vi "Main VI_1.vi"() -> ()   [LabVIEW 2024]
uses:
  Variable/Global.vi
  <vilib>/addons/database/Connection.llb/DB Tools Open Connec (String).vi
  <vilib>/addons/database/NI_Database_API.lvlib
  rpcrt4.dll
panel:
  out "String":string
  out "Config Path":path
  out "Communication error 3":bool
  out "Communication error 2":bool
  out "Communication error":bool
  in  "Logout 2":bool
  in  "USER TYPE":string(combo)="Admin"
  in  "USER NAME":string
  in  "PASSWORD":string
  in  "Login":bool
  out "Login Status":string
  in  "Calib":bool
  out "Login Type 2":string
  in  "Recipe":bool
  out "VER09042019":string
  out "Date Time":string
  in  "Manual":bool
  out "error out":errorcluster
  in  "Settings":bool
  in  "Report 2":bool
  in  "User_Setting":bool
  in  "Exit":bool
  in  "Run Test":bool
  out "User Name 2":string
  out "Login Type":string
  out "OK":bool
  # "TESTING DATALOGGING SYSTEM"
  # "31032025"
  # "SOFTWARE DEVELOPED BY:-SMOG Industries."
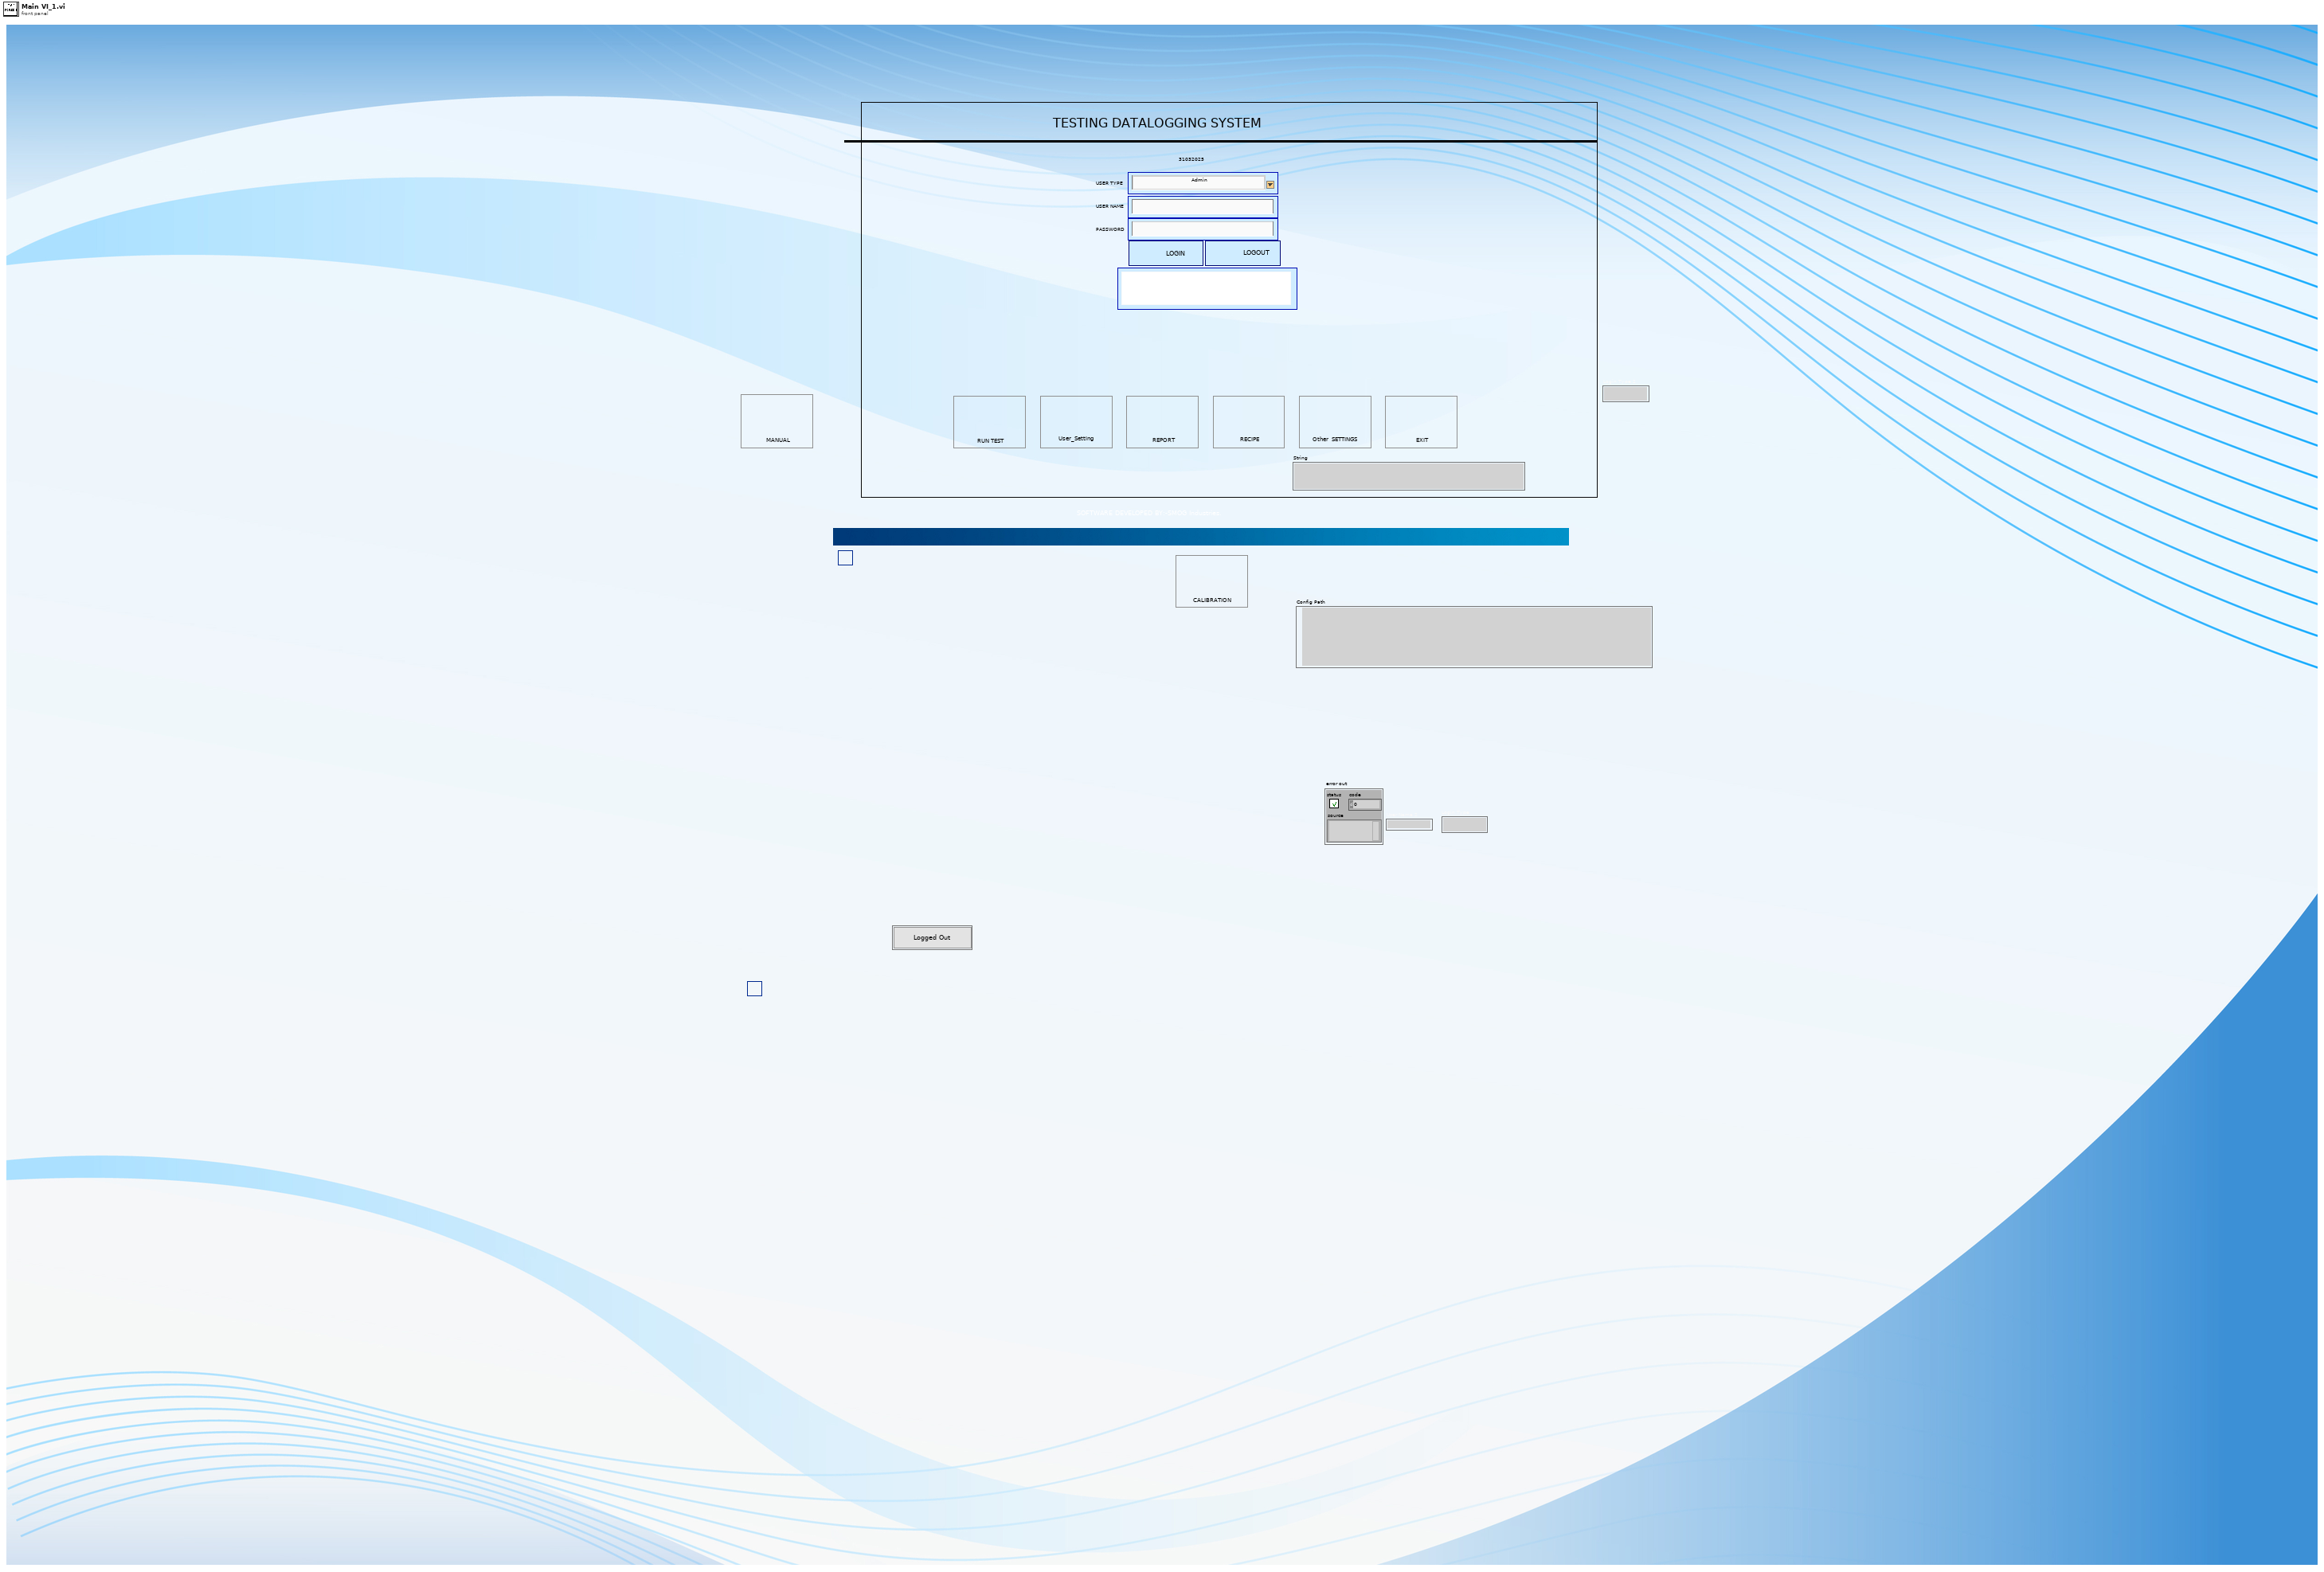
[diagram p1: front panel]
types:
  T1 = typedef "all path.ctl" = cluster{"User data":path, "Settings":path, "counter":path, "Test Setting":path, "IOs Path":path}
  T2 = enum16{"New barcode create", "barcode update", "check barcode", "database read", "barcode delete"}
  T3 = enum8{"Enabled", "Disabled", "Disabled and Grayed Out"}
  T4 = typedef "NI_Database_API.lvlib/Conn ObjectReference.ctl" = refnum<k1>
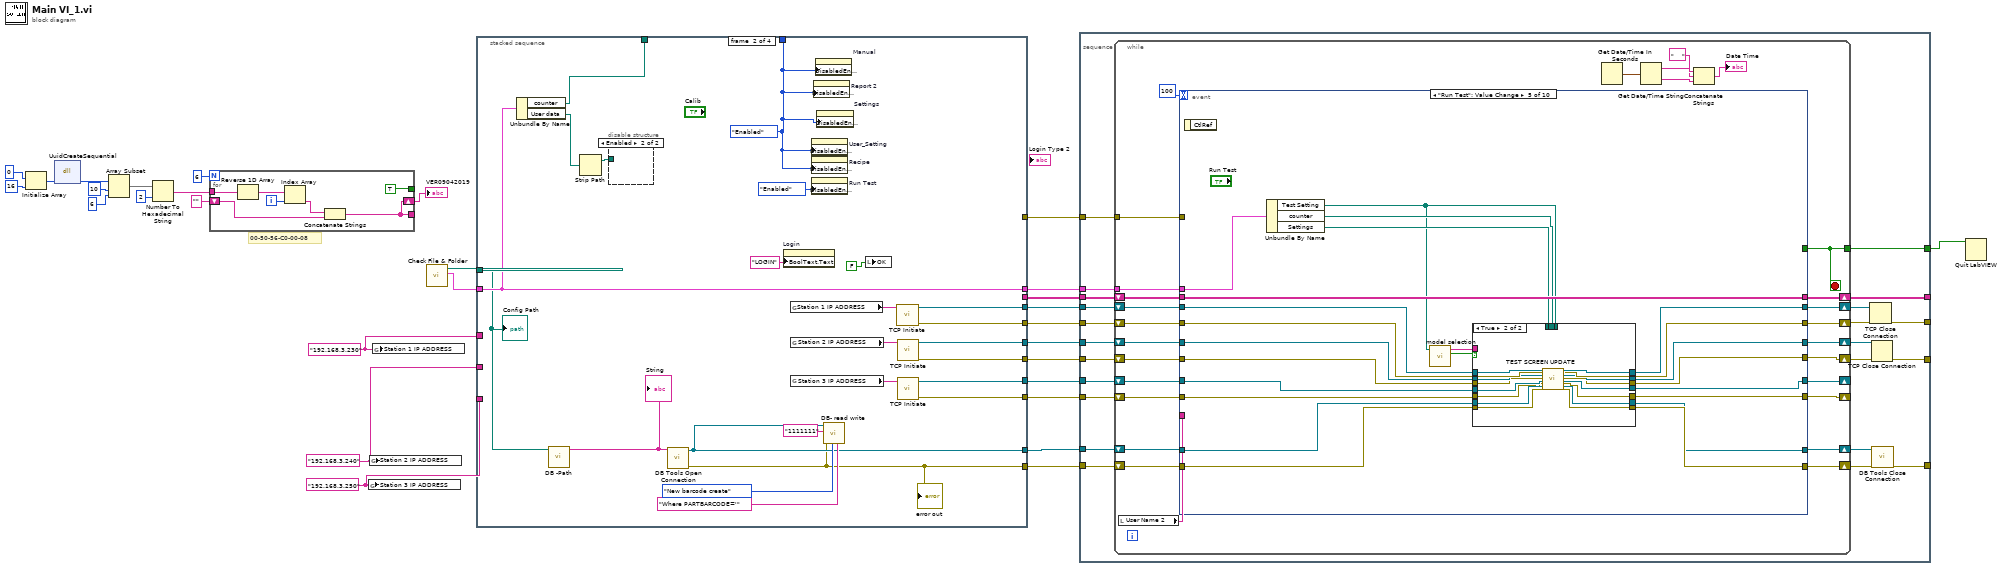
[diagram p0: block diagram]
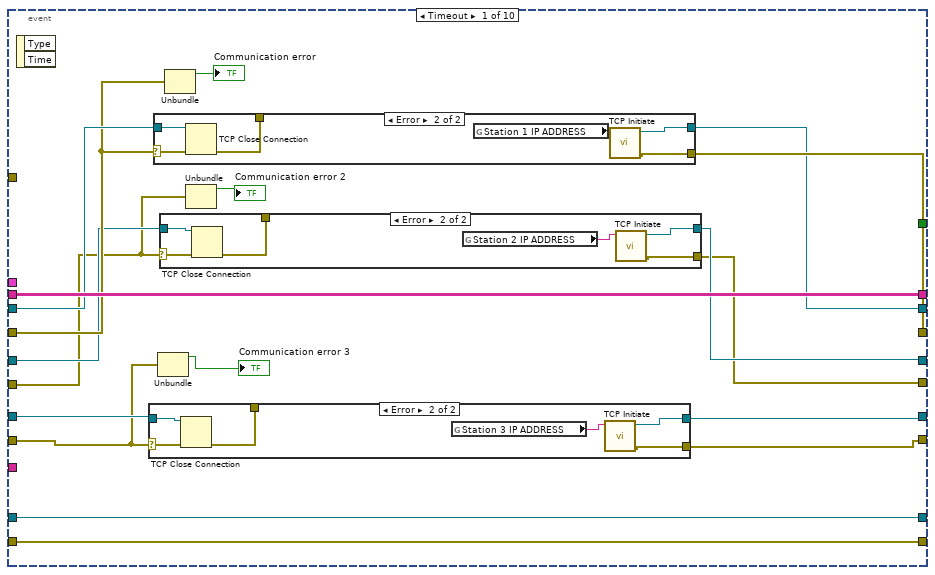
[diagram p2: hidden frame]
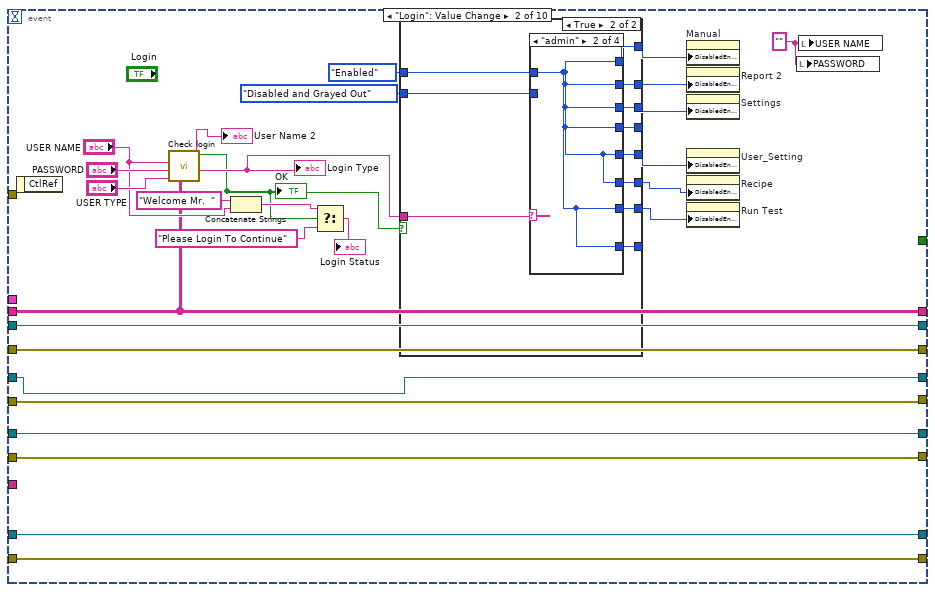
[diagram p6: hidden frame]
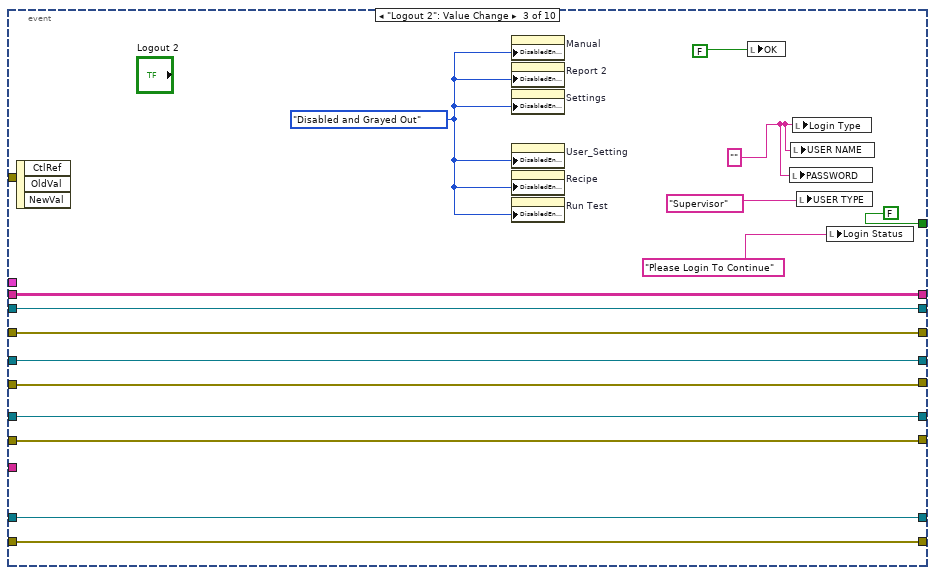
[diagram p11: hidden frame]
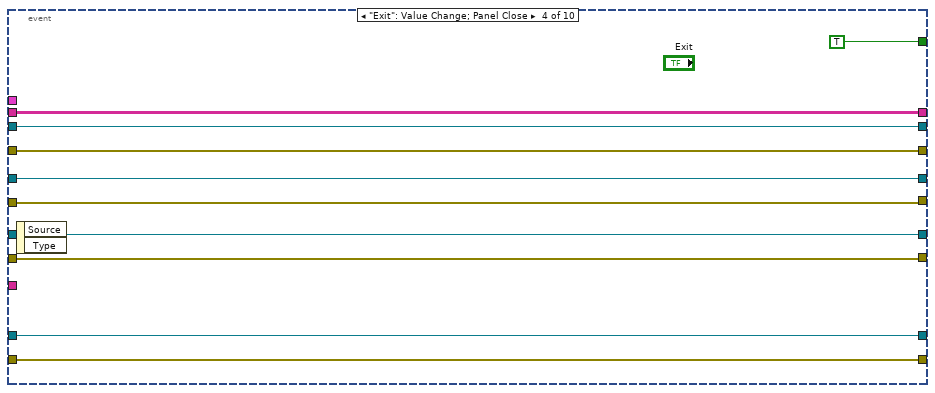
[diagram p12: hidden frame]
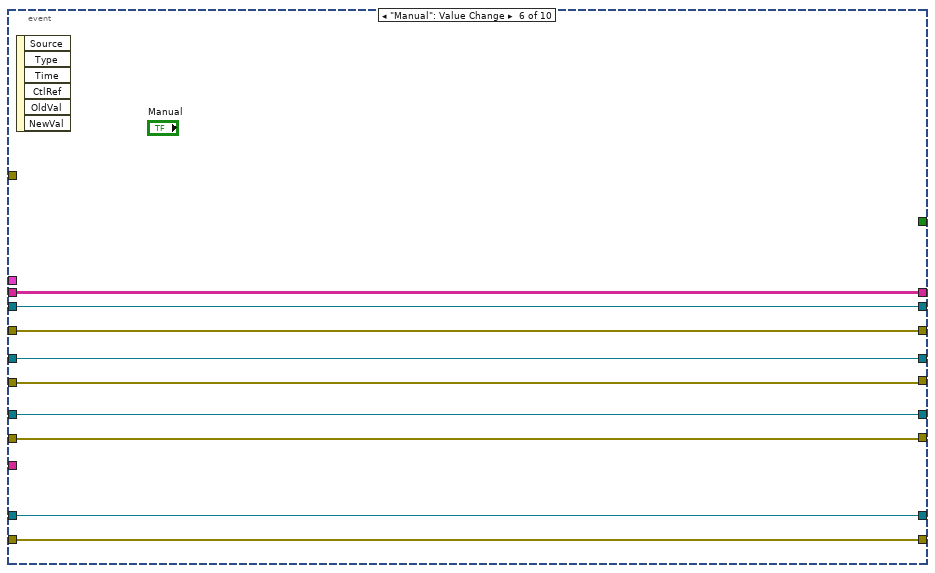
[diagram p14: hidden frame]
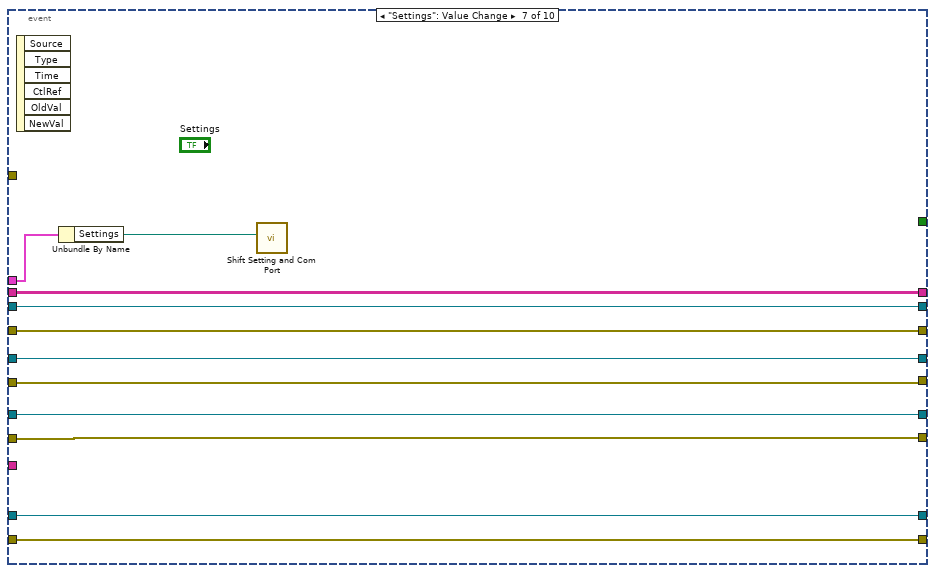
[diagram p15: hidden frame]
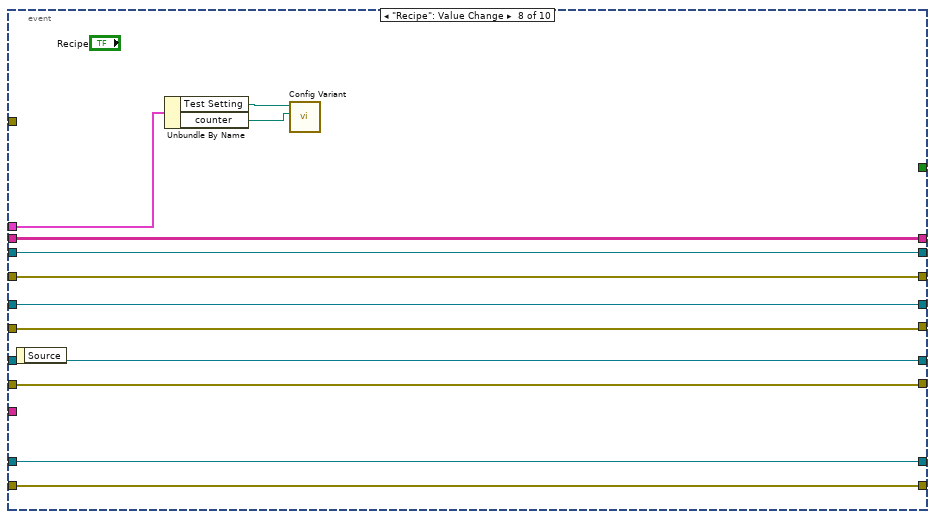
[diagram p16: hidden frame]
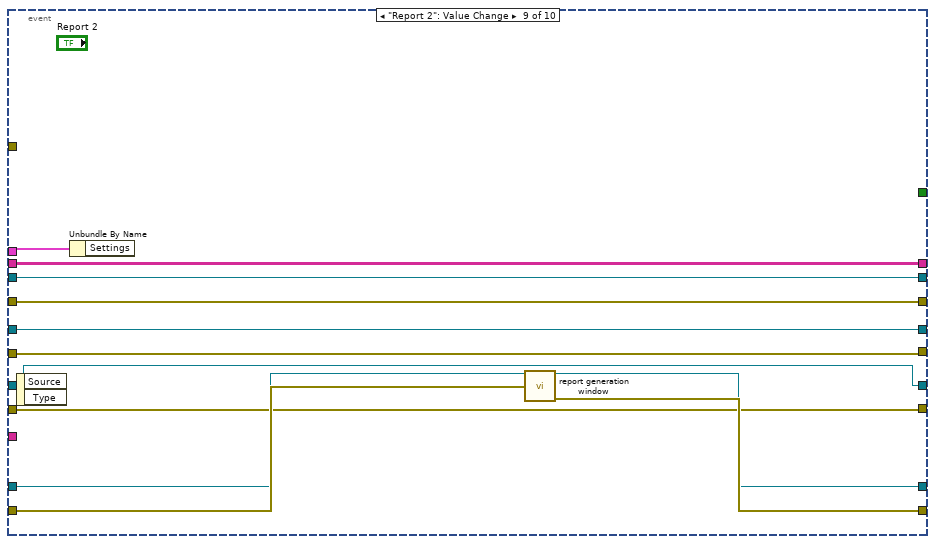
[diagram p17: hidden frame]
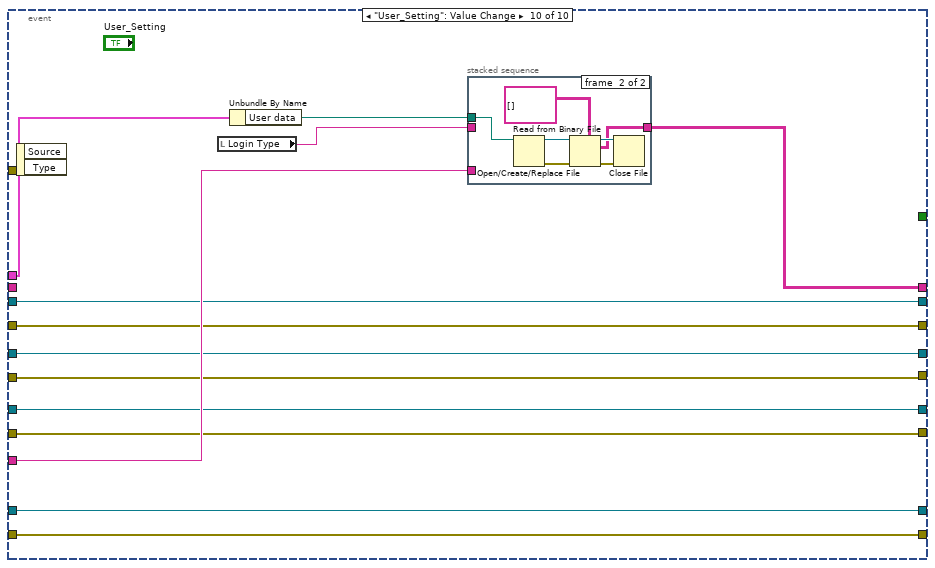
[diagram p18: hidden frame]
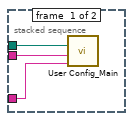
[diagram p19: hidden frame]
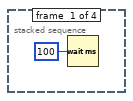
[diagram p20: hidden frame]
diagram:
  w3 = "192.168.3.250" ("LASER IP ADDRESS")
  w4 = "192.168.3.240" ("LASER IP ADDRESS")
  w5 = "192.168.3.230" ("LEAK IP ADDRESS")
  # "00-50-56-C0-00-08"
  n1 = Initialize Array(u8 0 ("uuid"), 16 ("dimension size")) -> (w11:u8[])
  n2 = dll-call lib="rpcrt4.dll" fn="UuidCreateSequential"("uuid"=w11) -> ("uuid"=w12:u8[])  [unwired: 4 in, 2 out]
  n3 = Array Subset(array=w12, index=10, length=6) -> (w13:u8[])
  n4 = Number To Hexadecimal String(1:i16 2 ("width (-)"), 2:w13) -> (0:w15:string[])
  n5 = for {
    N: 6 -> [_]
    tunnel: w15 -> [w32]
    shift-right: [w33] -> w8
    shift-left: "" -> [w34]
    tunnel: [w33] -> _
    tunnel: [TRUE] -> _
    i -> [w36]
    n6 = Reverse 1D Array(array=w32) -> (reversed array=w31:string[])
    n7 = Index Array(array=w31, index=w36) -> (element=w35:string)
    n8 = Concatenate Strings(w35, w34) -> (w33:string)
  }
  "VER09042019" <- w8
  n9 = global write "Global.vi" "Station 3 IP ADDRESS"(w3) -> ()
  n10 = global write "Global.vi" "Station 2 IP ADDRESS"(w4) -> ()
  n11 = global write "Global.vi" "Station 1 IP ADDRESS"(w5) -> ()
  n12 = call "Check File & Folder .vi"() -> ("Path 2"=w25:T1, "Config Path"=w26:path)  [unwired: 1 in, 9 out]
  n13 = stacked-sequence {
    tunnel: [_ _ w70 _] -> w29
    tunnel: w25 -> [_ w60 w68 _]
    tunnel: [_ _ w69 _] -> w28
    tunnel: [_ w60 _ _] -> w27
    tunnel: w26 -> [_ w38 _ _]
    tunnel: [_ w51 _ _] -> _
    tunnel: [_ w59 _ _] -> _
    tunnel: [_ w40 _ _] -> w23
    tunnel: [_ w39 _ _] -> w22
    tunnel: [_ w55 _ _] -> w21
    tunnel: [_ w54 _ _] -> w20
    tunnel: [_ w48 _ _] -> w7
    tunnel: [_ w47 _ _] -> w6
    tunnel: w5 -> [_ _ _ _]
    tunnel: w4 -> [_ _ _ _]
    tunnel: w3 -> [_ _ _ _]
    tunnel: [_ w45 _ _] -> w2
    tunnel: [_ w44 _ _] -> w1
    frame #0 {
      n14 = Wait (ms)(milliseconds to wait=u32 100) -> ()  [unwired: 1 out]
    }
    frame #1 {
      w51 = T3."Enabled" ("Disabled")
      n15 = Unbundle By Name(w60) -> ("counter"=w59:path, "User data"=w56:path)
      n16 = call "DB -Path.vi"("path"=w38) -> ("String"=w57:string)  [unwired: 8 in, 2 out]
      "String" <- w57
      n17 = Strip Path(path=w56) -> (stripped path=w53:path)  [unwired: 1 out]
      n18 = disable-structure shown="Enabled" {
        disable-tunnel: w53 -> [w62 _]
        frame Disabled {
          n19 = call "check license.vi"("created path"=w62) -> ()  [unwired: 11 in]
        }
        frame Enabled {
        }
      }
      n20 = call-poly <vilib>:"DB Tools Open Connection.vi"("connection information"=w57) -> ("error out"=w39:errorcluster, "connection reference"=w40:T4)  [unwired: 7 in]
      "error out" <- w39
      n21 = property on="Login" class="Bool"("BoolText.Text"="LOGIN" ("Boolean Text.Text")) -> ()  [unwired: 2 in, 2 out]
      n22 = global read "Global.vi" "Station 1 IP ADDRESS"() -> (w50:string)
      n23 = global read "Global.vi" "Station 2 IP ADDRESS"() -> (w49:string)
      n24 = global read "Global.vi" "Station 3 IP ADDRESS"() -> (w46:string)
      n25 = property on="User_Setting" class="Bool"("DisabledEnum"=w51) -> ()  [unwired: 2 in, 2 out]
      n26 = property on="Recipe" class="Bool"("DisabledEnum"=w51) -> ()  [unwired: 2 in, 2 out]
      n27 = property on="Run Test" class="Bool"("DisabledEnum"=T3."Enabled" ("Disabled")) -> ()  [unwired: 2 in, 2 out]
      n28 = property on="Report 2" class="Bool"("DisabledEnum"=w51) -> ()  [unwired: 2 in, 2 out]
      n29 = property on="Manual" class="Bool"("DisabledEnum"=w51) -> ()  [unwired: 2 in, 2 out]
      n30 = property on="Settings" class="Bool"("DisabledEnum"=w51) -> ()  [unwired: 2 in, 2 out]
      n31 = call "DB- read write.vi"("cmd"="Where PARTBARCODE='", "action"=T2."New barcode create", "error in (no error)"=w39, "BARCODE"="1111111", "connection reference"=w40) -> ()  [unwired: 3 in, 4 out]
      n32 = local write "OK"(FALSE ("result")) -> ()
      n33 = call "TCP Initiate.vi"("IP ADDRESS"=w50) -> ("error out"=w54:errorcluster, "connection ID"=w55:refnum<k5>)  [unwired: 9 in]
      n34 = call "TCP Initiate.vi"("IP ADDRESS"=w49) -> ("error out"=w47:errorcluster, "connection ID"=w48:refnum<k5>)  [unwired: 9 in]
      n35 = call "TCP Initiate.vi"("IP ADDRESS"=w46) -> ("error out"=w44:errorcluster, "connection ID"=w45:refnum<k5>)  [unwired: 9 in]
      "Config Path" <- w38
    }
    frame #2 {
      w65 = "" ("Password")
      n36 = call "validity.vi"() -> ("NOt valid"=w63:bool)  [unwired: 11 in]
      n37 = disable-structure shown="Enabled" {
        disable-tunnel: w63 -> [w77 _]
        frame Disabled {
          n38 = call "Prompt User for Input"("Enable"=w77) -> ("OK"=w76:bool)  [unwired: 17 in, 1 out]
          n39 = Quit LabVIEW(quit? (T)=w76) -> ()
        }
        frame Enabled {
        }
      }
      n40 = Unbundle By Name(w68) -> ("User data"=w67:path)
      n41 = Open/Create/Replace File(file path (use dialog)=w67) -> (refnum out=w74:refnum<file>, error out=w75:errorcluster)  [unwired: 5 in, 1 out]
      n42 = Read from Binary File(5:string[][] [] ("Cluster"), 8:w75, 11:w74) -> (0:w71:errorcluster, 2:w69:string[][], 3:w72:refnum<file>)  [unwired: 4 out]
      n43 = local write "Login Status"("Please Login To Continue" ("f")) -> ()
      n44 = local write "USER NAME"(w65) -> ()
      n45 = local write "PASSWORD"(w65) -> ()
      n46 = Close File(refnum=w72, error in=w71) -> (error out=w70:errorcluster)  [unwired: 1 out]
      n47 = local write "USER TYPE"("Supervisor" ("User Type")) -> ()
    }
    frame #3 {
      n48 = property on="USER NAME" class="Str"("Key Focus"=TRUE) -> ()  [unwired: 2 in, 2 out]
    }
  }
  n49 = stacked-sequence {
    tunnel: w29 -> [w100]
    tunnel: w28 -> [w99]
    tunnel: w27 -> [w98]
    tunnel: [w97] -> w24
    tunnel: [w96] -> _
    tunnel: w23 -> [w95]
    tunnel: w22 -> [w94]
    tunnel: [w91] -> _
    tunnel: w21 -> [w90]
    tunnel: w20 -> [w89]
    tunnel: [w86] -> _
    tunnel: w7 -> [w85]
    tunnel: w6 -> [w84]
    tunnel: [w81] -> _
    tunnel: w2 -> [w80]
    tunnel: w1 -> [w79]
    frame #0 {
      n50 = while {
        tunnel: w100 -> [w126]
        tunnel: w98 -> [w125]
        tunnel: [w124] -> w97
        shift-right: [w123] -> w96
        shift-left: w99 -> [w128]
        shift-right: [w113] -> w92
        shift-left: w94 -> [w115]
        shift-right: [w114] -> w93
        shift-left: w95 -> [w116]
        shift-right: [w109] -> w88
        shift-left: w90 -> [w112]
        shift-right: [w110] -> w87
        shift-left: w89 -> [w111]
        shift-right: [w106] -> w83
        shift-left: w85 -> [w108]
        shift-right: [w105] -> w82
        shift-left: w84 -> [w107]
        shift-right: [w104] -> _
        shift-left: w80 -> [w103]
        shift-right: [w102] -> _
        shift-left: w79 -> [w101]
        stop <- w124 stop-if-true
        n51 = local read "User Name 2"() -> (w122:string)
        n52 = event shown="[4] \"Run Test\": Value Change" {
          selector: _ -> [_ _ _ _ _ _ _ _ _ _]
          dyn-events: _ -> [_ _ _ _ _ _ _ _ _ _]
          timeout: 100 -> [_ _ _ _ _ _ _ _ _ _]
          tunnel: w128 -> [w146 w186 w228 w240 w264 w297 w308 w320 w332 _]
          tunnel: w126 -> [_ _ _ _ _ _ _ _ _ _]
          tunnel: w125 -> [_ _ _ _ w263 _ w307 w319 w325 w341]
          tunnel: [_ _ FALSE ("result") TRUE ("result") _ _ _ _ _ _] -> w124
          tunnel: [w146 w186 w228 w240 w264 w297 w308 w320 w332 w344] -> w123
          tunnel: w122 -> [_ _ _ _ _ _ _ _ _ w342]
          tunnel: w116 -> [w144 w183 w224 w238 w260 w296 w304 w316 w329 w339]
          tunnel: w115 -> [w145 w184 w225 w239 w262 w295 w305 w317 w331 w340]
          tunnel: [w144 w183 w224 w238 w259 w296 w304 w316 w328 w339] -> w114
          tunnel: [w145 w184 w225 w239 w261 w295 w305 w317 w330 w340] -> w113
          tunnel: w112 -> [w143 w181 w222 w236 w255 w293 w302 w314 w326 w337]
          tunnel: w111 -> [w139 w182 w223 w237 w258 w294 w303 w315 w327 w338]
          tunnel: [w142 w182 w223 w237 w256 w294 w303 w315 w327 w338] -> w110
          tunnel: [w141 w181 w222 w236 w254 w293 w302 w314 w326 w337] -> w109
          tunnel: w108 -> [w138 w174 w220 w235 w253 w292 w301 w312 w324 w336]
          tunnel: w107 -> [w134 w173 w219 w234 w252 w291 w300 w311 w323 w335]
          tunnel: [w137 w174 w220 w235 w251 w292 w301 w312 w324 w336] -> w106
          tunnel: [w136 w173 w219 w234 w250 w291 w300 w311 w323 w335] -> w105
          tunnel: [w133 w171 w217 w232 w243 w289 w299 w309 w321 w333] -> w104
          tunnel: w103 -> [w132 w171 w217 w232 w245 w289 w299 w309 w321 w333]
          tunnel: [w131 w172 w218 w233 w242 w290 w298 w310 w322 w334] -> w102
          tunnel: w101 -> [w130 w172 w218 w233 w244 w290 w298 w310 w322 w334]
          event Timeout {
            n53 = event-data() -> ()  [unwired: 3 out]
            n54 = case shown="Error" w130 {
              selector: w130 -> [w147 w154]
              tunnel: w132 -> [w148 w153]
              tunnel: [_ w152] -> _
              tunnel: [w148 w151] -> w133
              tunnel: [w147 w150] -> w131
              frame No Error {
              }
              frame Error {
                n55 = TCP Close Connection(connection ID=w153, error in (no error)=w154) -> (error out=w152:errorcluster)  [unwired: 1 in, 1 out]
                n56 = global read "Global.vi" "Station 3 IP ADDRESS"() -> (w149:string)
                n57 = call "TCP Initiate.vi"("IP ADDRESS"=w149) -> ("error out"=w150:errorcluster, "connection ID"=w151:refnum<k5>)  [unwired: 9 in]
              }
            }
            n58 = case shown="Error" w139 {
              selector: w139 -> [w163 w170]
              tunnel: w143 -> [w164 w169]
              tunnel: [_ w168] -> _
              tunnel: [w164 w167] -> w141
              tunnel: [w163 w166] -> w142
              frame No Error {
              }
              frame Error {
                n59 = TCP Close Connection(connection ID=w169, error in (no error)=w170) -> (error out=w168:errorcluster)  [unwired: 1 in, 1 out]
                n60 = global read "Global.vi" "Station 1 IP ADDRESS"() -> (w165:string)
                n61 = call "TCP Initiate.vi"("IP ADDRESS"=w165) -> ("error out"=w166:errorcluster, "connection ID"=w167:refnum<k5>)  [unwired: 9 in]
              }
            }
            n62 = Unbundle(w130) -> ("status"=→"Communication error 3":bool)  [unwired: 2 out]
            n63 = case shown="Error" w134 {
              selector: w134 -> [w155 w162]
              tunnel: w138 -> [w156 w161]
              tunnel: [_ w160] -> _
              tunnel: [w156 w159] -> w137
              tunnel: [w155 w158] -> w136
              frame No Error {
              }
              frame Error {
                n64 = TCP Close Connection(connection ID=w161, error in (no error)=w162) -> (error out=w160:errorcluster)  [unwired: 1 in, 1 out]
                n65 = global read "Global.vi" "Station 2 IP ADDRESS"() -> (w157:string)
                n66 = call "TCP Initiate.vi"("IP ADDRESS"=w157) -> ("error out"=w158:errorcluster, "connection ID"=w159:refnum<k5>)  [unwired: 9 in]
              }
            }
            n67 = Unbundle(w139) -> ("status"=→"Communication error":bool)  [unwired: 2 out]
            n68 = Unbundle(w134) -> ("status"=→"Communication error 2":bool)  [unwired: 2 out]
          }
          event "Login": Value Change {
            w198 = ""
            n69 = event-data() -> ()  [unwired: 2 out]
            n70 = call "Check login.vi"("Data I/p"=w186, "User Type"="USER TYPE", "Password"="PASSWORD", "User Name"="USER NAME") -> ("Login Type"=w194:string, "User Name 2"=→"User Name 2":string, "OK"=w185:bool)  [unwired: 2 in, 3 out]
            "OK" <- w185
            "Login Type" <- w194
            n71 = Concatenate Strings("Welcome Mr.  " ("string"), "USER NAME") -> (w195:string)
            n72 = Select(t=w195, s=w185, f="Please Login To Continue") -> (s? t:f=→"Login Status":string)
            n73 = case shown="True" w185 {
              tunnel: w194 -> [_ w210]
              tunnel: T3."Enabled" ("Disabled") -> [_ w209]
              tunnel: T3."Disabled and Grayed Out" ("f") -> [w199 w208]
              tunnel: [w199 w204] -> w176
              tunnel: [w199 w207] -> _
              tunnel: [w199 w206] -> w177
              tunnel: [w199 w205] -> w175
              tunnel: [w199 w203] -> w178
              tunnel: [w199 w202] -> w179
              tunnel: [w199 w201] -> w180
              tunnel: [w199 w200] -> _
              frame False {
              }
              frame True {
                n74 = case shown="\"admin\"" w210 {
                  tunnel: [w211 w212 w213 w215] -> w204
                  tunnel: w209 -> [_ w212 w214 w216]
                  tunnel: w208 -> [w211 _ w213 w215]
                  tunnel: [w211 w212 w214 w215] -> w207
                  tunnel: [w211 w212 w213 w215] -> w206
                  tunnel: [w211 w212 w214 w216] -> w205
                  tunnel: [w211 w212 w214 w215] -> w203
                  tunnel: [w211 w212 w214 w215] -> w202
                  tunnel: [w211 w212 w214 w215] -> w201
                  tunnel: [w211 w212 w214 w216] -> w200
                  frame "False", Default {
                  }
                  frame "admin" {
                  }
                  frame "super" {
                  }
                  frame "operator" {
                  }
                }
              }
            }
            n75 = property on="Manual" class="Bool"("DisabledEnum"=w180) -> ()  [unwired: 2 in, 2 out]
            n76 = property on="Report 2" class="Bool"("DisabledEnum"=w179) -> ()  [unwired: 2 in, 2 out]
            n77 = property on="Settings" class="Bool"("DisabledEnum"=w178) -> ()  [unwired: 2 in, 2 out]
            n78 = property on="User_Setting" class="Bool"("DisabledEnum"=w177) -> ()  [unwired: 2 in, 2 out]
            n79 = property on="Recipe" class="Bool"("DisabledEnum"=w176) -> ()  [unwired: 2 in, 2 out]
            n80 = property on="Run Test" class="Bool"("DisabledEnum"=w175) -> ()  [unwired: 2 in, 2 out]
            n81 = local write "PASSWORD"(w198) -> ()
            n82 = local write "USER NAME"(w198) -> ()
          }
          event "Logout 2": Value Change {
            w221 = T3."Disabled and Grayed Out" ("Disabled")
            w230 = "" ("Login Type")
            n83 = event-data() -> ()  [unwired: 4 out]
            n84 = property on="Manual" class="Bool"("DisabledEnum"=w221) -> ()  [unwired: 2 in, 2 out]
            n85 = property on="Report 2" class="Bool"("DisabledEnum"=w221) -> ()  [unwired: 2 in, 2 out]
            n86 = property on="Settings" class="Bool"("DisabledEnum"=w221) -> ()  [unwired: 2 in, 2 out]
            n87 = property on="User_Setting" class="Bool"("DisabledEnum"=w221) -> ()  [unwired: 2 in, 2 out]
            n88 = property on="Recipe" class="Bool"("DisabledEnum"=w221) -> ()  [unwired: 2 in, 2 out]
            n89 = property on="Run Test" class="Bool"("DisabledEnum"=w221) -> ()  [unwired: 2 in, 2 out]
            n90 = local write "OK"(FALSE ("OK")) -> ()
            n91 = local write "PASSWORD"(w230) -> ()
            n92 = local write "USER NAME"(w230) -> ()
            n93 = local write "Login Type"(w230) -> ()
            n94 = local write "USER TYPE"("Supervisor" ("User Type")) -> ()
            n95 = local write "Login Status"("Please Login To Continue" ("f")) -> ()
          }
          event "Exit": Value Change; Panel Close {
            n96 = event-data() -> ()  [unwired: 3 out]
          }
          event "Run Test": Value Change {
            n97 = event-data() -> ()  [unwired: 2 out]
            n98 = Unbundle By Name(w263) -> ("Test Setting"=w246:path, "counter"=w249:path, "Settings"=w257:path)
            n99 = call "model selection.vi"("file path (use dialog)"=w246) -> ("OK"=w248:bool, "Test Name 2"=w247:string)  [unwired: 9 in]
            n100 = case shown="True" w248 {
              tunnel: w262 -> [w267 w288]
              tunnel: [w267 w287] -> w261
              tunnel: w260 -> [w268 w286]
              tunnel: [w268 w285] -> w259
              tunnel: w258 -> [w271 w284]
              tunnel: w257 -> [_ _]
              tunnel: [w271 w283] -> w256
              tunnel: w255 -> [w272 w282]
              tunnel: [w272 w281] -> w254
              tunnel: w253 -> [w270 w280]
              tunnel: w252 -> [w269 w279]
              tunnel: [w270 w278] -> w251
              tunnel: [w269 w277] -> w250
              tunnel: w246 -> [_ _]
              tunnel: w249 -> [_ _]
              tunnel: w247 -> [_ _]
              tunnel: w245 -> [w266 w276]
              tunnel: w244 -> [w265 w275]
              tunnel: [w266 w274] -> w243
              tunnel: [w265 w273] -> w242
              frame False {
              }
              frame True {
                n101 = call "TEST SCREEN UPDATE.vi"("Staion  in 1"=w282, "Staion  in 2"=w280, "Staion  in error 2"=w279, "Staion  in 3"=w276, "Staion  in error 3"=w275, "DataBase connection in"=w286, "Database error in"=w288, "Staion  in error 1"=w284) -> ("Staion Error Out 1"=w283:errorcluster, "Staion Out 1"=w281:refnum<k5>, "Staion Out 2"=w278:refnum<k5>, "Staion Error Out 2"=w277:errorcluster, "Staion Out 3"=w274:refnum<k5>, "Staion Error Out 3"=w273:errorcluster, "Database connection out"=w285:T4, "Database error out"=w287:errorcluster)  [unwired: 12 in]
              }
            }
          }
          event "Manual": Value Change {
            n102 = event-data() -> ()  [unwired: 7 out]
          }
          event "Settings": Value Change {
            n103 = event-data() -> ()  [unwired: 7 out]
            n104 = Unbundle By Name(w307) -> ("Settings"=w306:path)
            n105 = call "Shift Setting and Com Port.vi"("Setting"=w306) -> ()  [unwired: 10 in, 1 out]
          }
          event "Recipe": Value Change {
            n106 = event-data() -> ()  [unwired: 2 out]
            n107 = Unbundle By Name(w319) -> ("Test Setting"=w318:path, "counter"=w313:path)
            n108 = call "Config Variant.vi"("Count"=w313, "test sequence"=w318) -> ()  [unwired: 10 in]
          }
          event "Report 2": Value Change {
            n109 = event-data() -> ()  [unwired: 3 out]
            n110 = Unbundle By Name(w325) -> ()  [unwired: 1 out]
            n111 = call "report generation  window.vi"("connection reference"=w329, "error in"=w331) -> ("connection reference out"=w328:T4, "error out"=w330:errorcluster)  [unwired: 12 in]
          }
          event "User_Setting": Value Change {
            n112 = event-data() -> ()  [unwired: 3 out]
            n113 = local read "Login Type"() -> (w343:string)
            n114 = Unbundle By Name(w341) -> ("User data"=w345:path)
            n115 = stacked-sequence {
              tunnel: w345 -> [w348 w350]
              tunnel: [_ w349] -> w344
              tunnel: w343 -> [w347 _]
              tunnel: w342 -> [w346 _]
              frame #0 {
                n116 = call "User Config_Main.vi"("Login Status"=w346, "User Type"=w347, "Path"=w348) -> ()  [unwired: 9 in]
              }
              frame #1 {
                n117 = Open/Create/Replace File(file path (use dialog)=w350) -> (refnum out=w352:refnum<file>, error out=w351:errorcluster)  [unwired: 5 in, 1 out]
                n118 = Read from Binary File(5:string[][] [] ("Cluster"), 8:w351, 11:w352) -> (0:w355:errorcluster, 2:w349:string[][], 3:w354:refnum<file>)  [unwired: 4 out]
                n119 = Close File(refnum=w354, error in=w355) -> ()  [unwired: 2 out]
              }
            }
          }
        }
        n120 = Get Date/Time In Seconds() -> (seconds since 1Jan1904=w121:timestamp)
        n121 = Get Date/Time String(seconds (now)=w121) -> (date string=w120:string, time string=w119:string)  [unwired: 2 in]
        n122 = Concatenate Strings(w120, "    " ("string"), w119) -> (→"Date Time":string)
      }
      n123 = TCP Close Connection(connection ID=w88, error in (no error)=w87) -> (error out=w86:errorcluster)  [unwired: 1 in, 1 out]
      n124 = TCP Close Connection(connection ID=w83, error in (no error)=w82) -> (error out=w81:errorcluster)  [unwired: 1 in, 1 out]
      n125 = call <vilib>:"DB Tools Close Connection.vi"("error in (no error)"=w92, "connection reference"=w93) -> ("error out"=w91:errorcluster)  [unwired: 5 in]
    }
  }
  n126 = Quit LabVIEW(quit? (T)=w24) -> ()
